vi "Search_Array.vi"(8 "Search":dbl, 11 "Array":dbl[](array[numeric])) -> (1 "Index":i32)   [LabVIEW 2022 SP3]
panel:
  out "Found?":bool
  # "Search_Array:\nPopulate the blank array below, and enter a value to search for.\nIf the value is found in the array. its index will be displayed along\nwith a lit LED light. If it is not found, the index of -1 will be displayed."
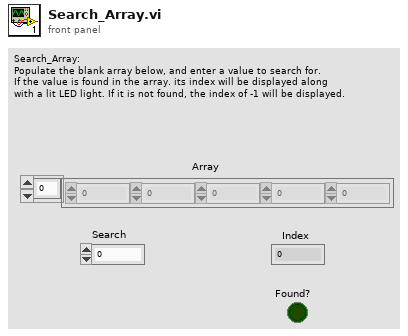
[diagram p1: front panel]
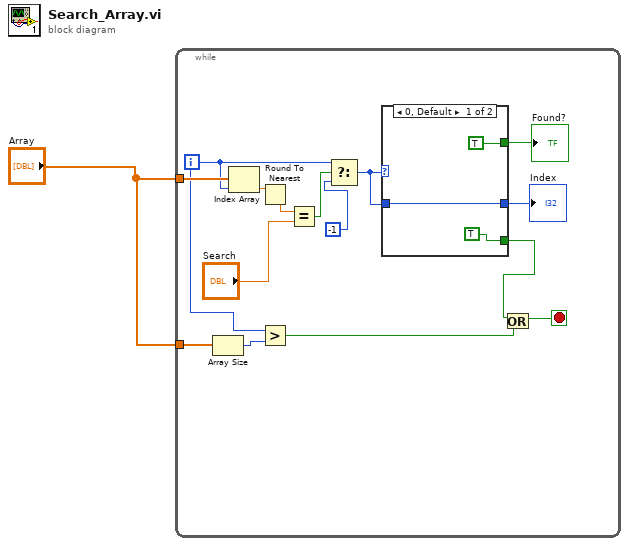
[diagram p0: block diagram]
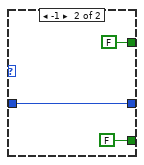
[diagram p2: hidden frame]
diagram:
  n1 = while {
    tunnel: "Array" -> [w16]
    tunnel: "Array" -> [w3]
    i -> [w7]
    stop <- w5 stop-if-true
    n2 = Array Size(array=w3) -> (size(s)=w8:i32)
    n3 = Index Array(array=w16, index=w7) -> (element=w14:dbl)
    n4 = Round To Nearest(number=w14) -> (nearest integer value=w2:dbl)
    n5 = Greater?(x=w7, y=w8) -> (0:w6:bool)
    n6 = Equal?(x=w2, y="Search") -> (x = y?=w13:bool)
    n7 = Select(t=w7, s=w13, f=-1) -> (s? t:f=w11:i32)
    n8 = case shown="0, Default" w11 {
      tunnel: w11 -> [w19 w22]
      tunnel: [w19 w22] -> w10
      tunnel: [TRUE FALSE] -> w4
      tunnel: [TRUE FALSE] -> w9
      frame 0, Default {
      }
      frame -1 {
      }
    }
    "Index" <- w10
    "Found?" <- w9
    n9 = Or(x=w4, y=w6) -> (x .or. y?=w5:bool)
  }
